vi "Write m.vi"(8 "error in (no error)":errorcluster, 10 "m":dbl, 11 "RFID system in":refnum<class "RFID system.lvclass">) -> (0 "error out":errorcluster, 3 "RFID system out":refnum<class "RFID system.lvclass">)   [LabVIEW 2019, in "RFID system.lvclass"]
uses:
  RFID system.lvclass
  RFID system.lvclass/RFID system.ctl
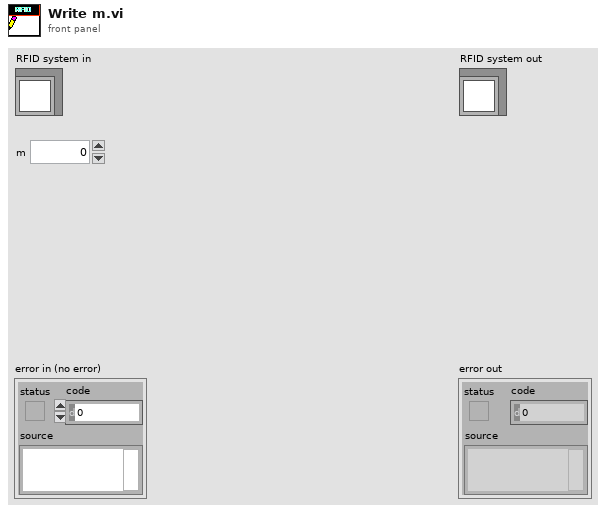
[diagram p1: front panel]
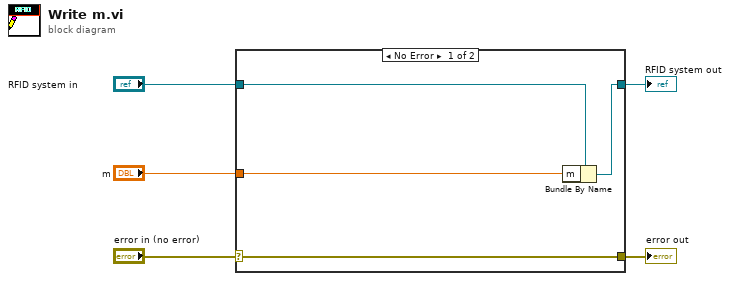
[diagram p0: block diagram]
diagram:
  n1 = case shown="No Error" "error in (no error)" {
    selector: "error in (no error)" -> [w9 w10]
    tunnel: [w9 w10] -> w4
    tunnel: [w7 w11] -> w2
    tunnel: "RFID system in" -> [w8 w11]
    tunnel: "m" -> [w6 _]
    frame No Error {
      n2 = Bundle By Name(cluster=w8, "m"=w6) -> (w7:refnum<class "RFID system.lvclass">)
    }
    frame Error {
    }
  }
  "error out" <- w4
  "RFID system out" <- w2
